vi "CommandR.vi"(0 "RBD9103":T2, 2 "Operation":T1, 3 "Command":string, 4 "Data":string, 5 "error in":errorcluster) -> (11 "Command time, ms":u32, 14 "RBD9103 out":T2, 16 "Answer":string, 19 "error out":errorcluster)   [LabVIEW 2018]
uses:
  RBD9103.ctl
  GenericDataEvent/GenericEvent.ctl
  Operation type.ctl
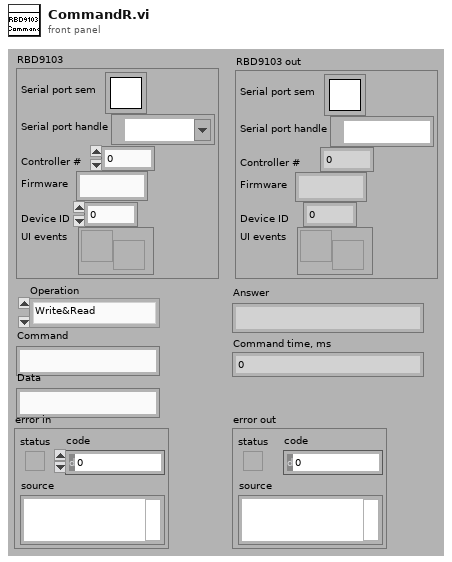
[diagram p1: front panel]
types:
  T1 = typedef "Operation type.ctl" = enum16{"Write&Read", "Read only", "Write only", "Read only multiply"}
  T2 = typedef "RBD9103.ctl" = cluster{"Serial port sem":T3, "Serial port handle":refnum<visa-resource-name>, "Controller #":u8, "Firmware":string, "Device ID":i32, "UI events":T4}
  T3 = typedef "Semaphore RefNum" = refnum<k1>
  T4 = typedef "GenericEvent.ctl" = refnum<user-event>
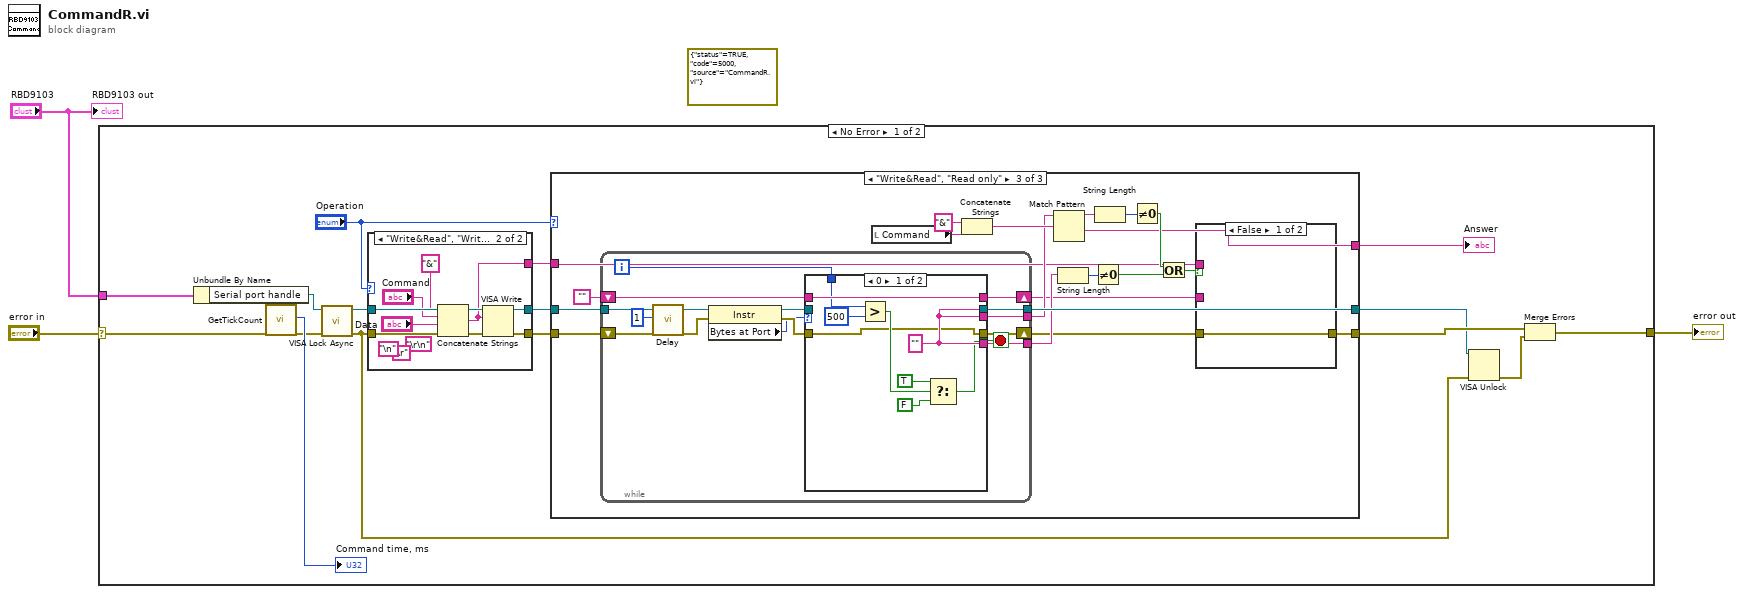
[diagram p0: block diagram]
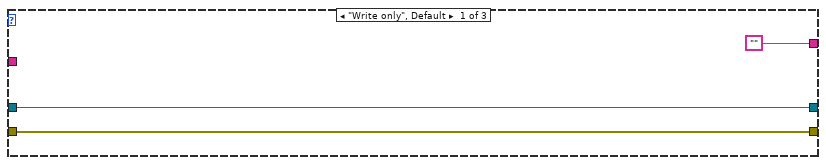
[diagram p2: hidden frame]
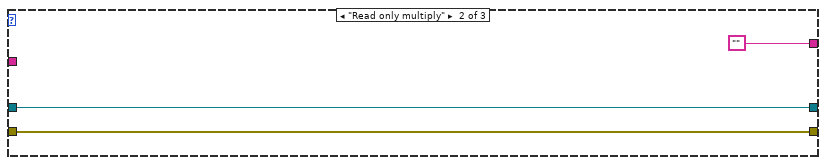
[diagram p3: hidden frame]
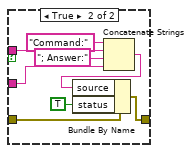
[diagram p4: hidden frame]
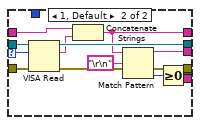
[diagram p5: hidden frame]
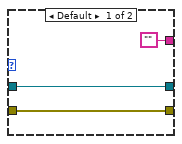
[diagram p6: hidden frame]
diagram:
  (unwired) errorcluster {"status"=TRUE, "code"=5000, "source"="CommandR.vi"} ("error out")
  n1 = case shown="No Error" "error in" {
    selector: "error in" -> [w11 w104]
    tunnel: [w19 w104] -> w2
    tunnel: "RBD9103" -> [w18 _]
    frame No Error {
      n2 = Unbundle By Name(w18) -> ("Serial port handle"=w14:refnum<visa-resource-name>)
      n3 = call "GetTickCount.vi"("error in (no error)"=w11) -> ("ms"=→"Command time, ms":u32, "error IO"=w12:errorcluster)  [unwired: 17 in]
      n4 = call <vilib>:"VISA Lock Async.vi"("error in (no error)"=w12, "VISA resource name"=w14) -> ("error out"=w10:errorcluster, "VISA resource name out"=w13:refnum<visa-resource-name>)  [unwired: 7 in, 1 out]
      n5 = case shown="\"Write&Read\", \"Write only\"" "Operation" {
        tunnel: w13 -> [w94 w103]
        tunnel: [w94 w102] -> w17
        tunnel: [w93 w101] -> w16
        tunnel: w10 -> [w93 w100]
        tunnel: ["" w96] -> w5
        frame Default {
        }
        frame "Write&Read", "Write only" {
          (unwired) "\r"
          (unwired) "\n"
          n6 = Concatenate Strings("&" ("string"), "Command", "Data", "\r\n") -> (w96:string)
          n7 = VISA Write(VISA resource name=w103, write buffer=w96, error in (no error)=w100) -> (VISA resource name out=w102:refnum<visa-resource-name>, error out=w101:errorcluster)  [unwired: 1 out]
        }
      }
      n8 = case shown="\"Write&Read\", \"Read only\"" "Operation" {
        tunnel: w17 -> [w21 w24 w45]
        tunnel: w16 -> [w22 w25 w44]
        tunnel: [w22 w25 w30] -> w8
        tunnel: [w21 w24 w43] -> w6
        tunnel: w5 -> [_ _ w29]
        tunnel: ["" "" w33] -> w4
        frame "Write only", Default {
        }
        frame "Read only multiply" {
        }
        frame "Write&Read", "Read only" {
          n9 = while {
            tunnel: w45 -> [w68]
            shift-right: [w65] -> w31
            shift-left: w44 -> [w58]
            tunnel: [w64] -> w43
            tunnel: [w63] -> w39
            tunnel: [w62] -> w37
            shift-right: [w60] -> w28
            shift-left: "" -> [w61]
            i -> [w55]
            stop <- w66 stop-if-true
            n10 = call "Delay.vi"("Delay, ms"=u32 1, "error in"=w58) -> ("error out"=w57:errorcluster)  [unwired: 17 in]
            n11 = property class="Instr"(reference=w68, error in=w57) -> (reference out=w67:refnum<visa-resource-name>, error out=w69:errorcluster, "Bytes at Port"=w59:u32)
            n12 = case shown="0" w59 {
              selector: w59 -> [_ w79]
              tunnel: w69 -> [w73 w91]
              tunnel: w67 -> [_ w90]
              tunnel: [w71 w87] -> w66
              tunnel: [w73 w86] -> w65
              tunnel: [w77 w85] -> w64
              tunnel: [w77 w84] -> w63
              tunnel: [w77 w83] -> w62
              tunnel: w61 -> [w78 w82]
              tunnel: [w78 w80] -> w60
              tunnel: w55 -> [w76 _]
              frame 0 {
                w77 = ""
                n13 = Greater?(x=w76, y=500) -> (0:w74:bool)
                n14 = Select(t=TRUE, s=w74, f=FALSE) -> (s? t:f=w71:bool)
              }
              frame 1, Default {
                n15 = VISA Read(VISA resource name=w90, byte count=w79, error in (no error)=w91) -> (VISA resource name out=w85:refnum<visa-resource-name>, read buffer=w81:string, error out=w86:errorcluster)  [unwired: 1 out]
                n16 = Concatenate Strings(w82, w81) -> (w80:string)
                n17 = Match Pattern(string=w80, regular expression="\r\n") -> (before substring=w84:string, after substring=w83:string, offset past match=w88:i32)  [unwired: 1 in, 1 out]
                n18 = Greater Or Equal To 0?(x=w88) -> (x >= 0?=w87:bool)
              }
            }
          }
          n19 = local read "Command"() -> (w41:string)
          n20 = Concatenate Strings("&" ("string"), w41) -> (w42:string)
          n21 = Match Pattern(string=w39, regular expression=w42) -> (before substring=w27:string, after substring=w33:string)  [unwired: 1 in, 2 out]
          n22 = String Length(string=w37) -> (length=w38:i32)
          n23 = Not Equal To 0?(x=w38) -> (x != 0?=w35:bool)
          n24 = String Length(string=w27) -> (length=w26:i32)
          n25 = Not Equal To 0?(x=w26) -> (x != 0?=w34:bool)
          n26 = Or(x=w34, y=w35) -> (x .or. y?=w32:bool)
          n27 = case shown="False" w32 {
            tunnel: w31 -> [w46 w53]
            tunnel: [w46 w54] -> w30
            tunnel: w29 -> [_ w50]
            tunnel: w28 -> [_ w48]
            frame False {
            }
            frame True {
              n28 = Concatenate Strings("Command:" ("string"), w50, "; Answer:" ("string"), w48) -> (w47:string)
              n29 = Bundle By Name(cluster=w53, "source"=w47, "status"=TRUE) -> (w54:errorcluster)
            }
          }
        }
      }
      "Answer" <- w4
      n30 = VISA Unlock(8:w10, 11:w6) -> (0:w9:errorcluster)  [unwired: 1 out]
      n31 = Merge Errors(w8, w9) -> (w19:errorcluster)
    }
    frame Error {
    }
  }
  "error out" <- w2
  "RBD9103 out" <- "RBD9103"
